vi "Set Buttons States.vi"(8 "error in (no error)":errorcluster, 9 "Button States":T1[](array[typedef]), 10 "Button Indexes":i32[](array[numeric]), 11 "Toolbar Control in":refnum<class "Toolbar Control.lvclass">) -> (0 "error out":errorcluster, 2 "Toolbar Image":picture, 3 "Toolbar Control out":refnum<class "Toolbar Control.lvclass">)   [LabVIEW 2011, in "Toolbar Control.lvclass"]
doc: "This VI sets the buttons specified by their indexes <B>Button Indexes</B> to the states <B>Button States</B>. If <B>Button States</B> is not provided they default to enabled.\n\n-------------\nDeveloped by Brian Hoover (hooovahh)"
uses:
  Toolbar Control.lvclass
  Controls/Button State.ctl
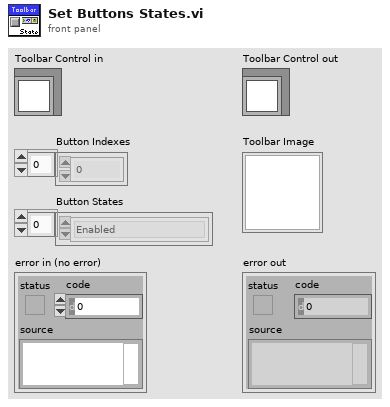
[diagram p1: front panel]
types:
  T1 = typedef "Toolbar Control.lvclass/Button State.ctl" = enum8{"Enabled", "Disabled", "Disabled and Grayed Out"}
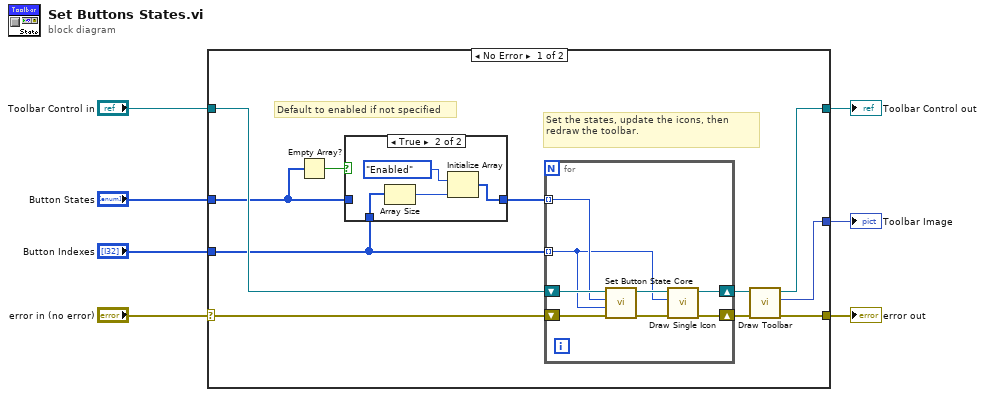
[diagram p0: block diagram]
diagram:
  n1 = case shown="No Error" "error in (no error)" {
    selector: "error in (no error)" -> [w16 w33]
    tunnel: [w15 w33] -> w6
    tunnel: [w13 w32] -> w4
    tunnel: "Toolbar Control in" -> [w14 w32]
    tunnel: "Button States" -> [w11 _]
    tunnel: "Button Indexes" -> [w9 _]
    tunnel: [w8 _] -> w1
    frame No Error {
      # "Set the states, update the icons, then redraw the toolbar."
      # "Default to enabled if not specified"
      n2 = Empty Array?(array=w11) -> (empty?=w12:bool)
      n3 = case shown="True" w12 {
        tunnel: w11 -> [w19 _]
        tunnel: [w19 w20] -> w10
        tunnel: w9 -> [_ w22]
        frame False {
        }
        frame True {
          n4 = Array Size(array=w22) -> (size(s)=w21:i32)
          n5 = Initialize Array(Button_State."Enabled" ("Button State"), w21) -> (w20:T1[])
        }
      }
      n6 = for {
        shift-right: [w30] -> w17
        shift-left: w14 -> [w26]
        shift-right: [w31] -> w18
        shift-left: w16 -> [w27]
        tunnel: w10 -> [w25] mode=indexing
        tunnel: w9 -> [w24] mode=indexing
        n7 = call "Set Button State Core.vi"("error in (no error)"=w27, "Button Index"=w24, "Button State"=w25, "Toolbar Control in"=w26) -> ("error out"=w28:errorcluster, "Toolbar Control out"=w29:refnum<class "Toolbar Control.lvclass">)  [unwired: 6 in]
        n8 = call "Draw Single Icon.vi"("error in (no error)"=w28, "Icon Index"=w24, "Toolbar Control in"=w29) -> ("error out"=w31:errorcluster, "Toolbar Control out"=w30:refnum<class "Toolbar Control.lvclass">)  [unwired: 7 in]
      }
      n9 = call "Draw Toolbar.vi"("error in (no error)"=w18, "Toolbar Control in"=w17) -> ("error out"=w15:errorcluster, "Toolbar Image"=w8:picture, "Toolbar Control out"=w13:refnum<class "Toolbar Control.lvclass">)  [unwired: 7 in]
    }
    frame Error {
    }
  }
  "error out" <- w6
  "Toolbar Control out" <- w4
  "Toolbar Image" <- w1
